vi "RT Test.vi"(11 "Data In":T1) -> (3 "Data Out":T1)   [LabVIEW 2016]
doc: "Assert Component\nAssert Name: RT Test\nData Type: Double Float\nDeveloped by UKHornP\nEvaluation String: X > 1.500000\nDescription: Who knows?"
uses:
  Core/Assert API Components/Assert API Components.lvlib
  Core/Assert API Components/VI References.ctl
  Core/Assert API Components/Failure Actions.ctl
  Plugins/Templates/NC Templates/dbl.ctl
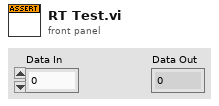
[diagram p1: front panel]
types:
  T1 = typedef "dbl.ctl" = dbl
  T2 = typedef "Assert API Components.lvlib/VI References.ctl" = cluster{"Calling VI Ref":refnum<vi>, "Assert VI Ref":refnum<vi>}
  T3 = typedef "Assert API Components.lvlib/Failure Actions.ctl" = enum16{"None", "Log To File", "Pause Execution", "Abort Execution"}
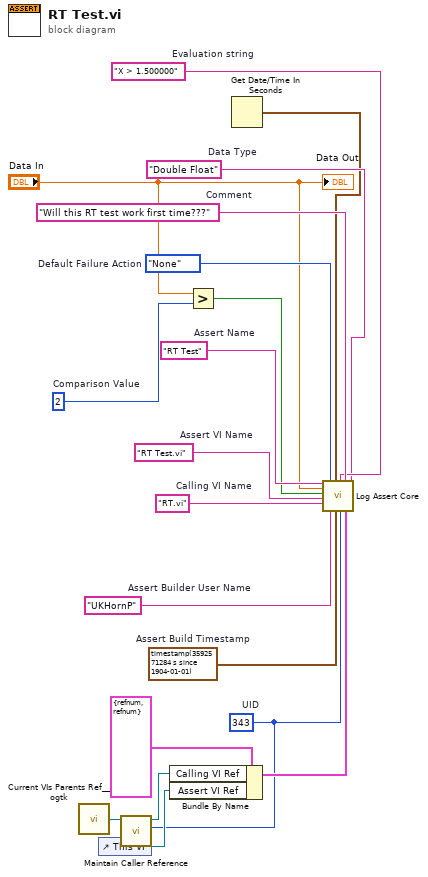
[diagram p0: block diagram]
diagram:
  w1 = 343  # UID
  w4 = "RT Test.vi"  # Assert VI Name
  w5 = "RT.vi"  # Calling VI Name
  w6 = timestamp(3592571284.2530556 s since 1904-01-01)  # Assert Build Timestamp
  w7 = "UKHornP"  # Assert Builder User Name
  w8 = "Double Float"  # Data Type
  w16 = "Will this RT test work first time???"  # Comment
  w13 = "X > 1.500000"  # Evaluation string
  w18 = Failure_Actions."None"  # Default Failure Action
  w19 = "RT Test"  # Assert Name
  w17 = 2  # Comparison Value
  n1 = call <userlib>:"Current VIs Parents Ref__ogtk.vi"() -> ("Calling VI's Reference"=w11:refnum<vi>)  [unwired: 2 in]
  n2 = control-ref of="This VI"() -> (w10:refnum<vi>)
  n3 = call "Maintain Caller Reference.vi"("UID"=w1, "VI in"=w11) -> ("VI out"=w3:refnum<vi>)  [unwired: 9 in]
  n4 = Bundle By Name(cluster=T2 {"Calling VI Ref"=refnum, "Assert VI Ref"=refnum} ("VI References"), "Calling VI Ref"=w3, "Assert VI Ref"=w10) -> (w9:T2)
  n5 = Greater?(x="Data In", y=w17) -> (0:w14:bool)
  n6 = Get Date/Time In Seconds() -> (seconds since 1Jan1904=w2:timestamp)
  n7 = call "Log Assert Core.vi"("Assert Name"=w19, "Data Value"="Data In", "Status"=w14, "Assert VI Name"=w4, "Calling VI Name"=w5, "Failure Action"=w18, "Assert Builder User Name"=w7, "Last Update"=w2, "Assert Build Timestamp"=w6, "Evaluation String"=w13, "Assert VI UID"=w1, "Comment"=w16, 13:w9, "Data Type"=w8) -> ()  [unwired: 6 in]
  "Data Out" <- "Data In"
